vi "Two_Functions.vi"() -> ()   [LabVIEW 2022 SP3]
panel:
  out "Answer":dbl
  out "g(x,y) = 4x + 5y":bool
  out "f(x,y) = 2x + 3y":bool
  in  "y":dbl
  in  "x":dbl
  # "Two_Functions:\nBegin by entering a value for x and y.\nIf x > y, f(x,y) will be computed. If x < y,\ng(x,y) will be computed."
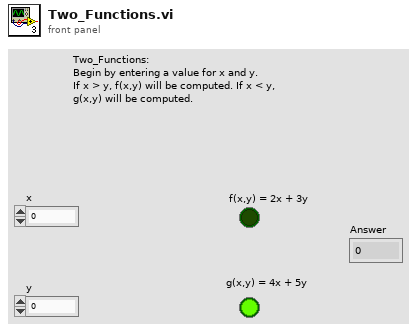
[diagram p1: front panel]
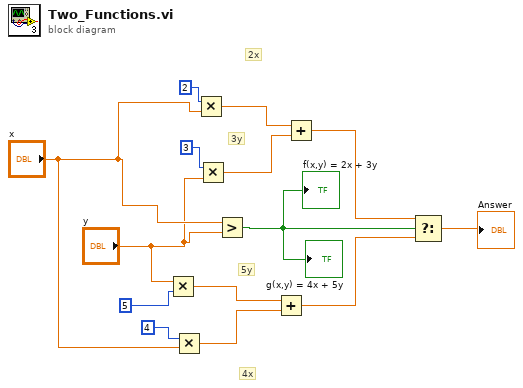
[diagram p0: block diagram]
diagram:
  # "3y"
  # "2x"
  # "4x"
  # "5y"
  n1 = Multiply(x="y", y=5) -> (x*y=w8:dbl)
  n2 = Multiply(x=4, y="x") -> (x*y=w7:dbl)
  n3 = Multiply(x=2, y="x") -> (x*y=w13:dbl)
  n4 = Multiply(x=3, y="y") -> (x*y=w11:dbl)
  n5 = Greater?(x="x", y="y") -> (0:w1:bool)
  "f(x,y) = 2x + 3y" <- w1
  "g(x,y) = 4x + 5y" <- w1
  n6 = Add(x=w8, y=w7) -> (x+y=w3:dbl)
  n7 = Add(x=w13, y=w11) -> (x+y=w4:dbl)
  n8 = Select(t=w4, s=w1, f=w3) -> (s? t:f=→"Answer":dbl)
